vi "WS2812 Ring LED.vi"() -> ()   [LabVIEW 2017]
uses:
  IMAQCV/PIIO/Core/PIIO DIO.ctl
  IMAQCV/PIIO.lvlib
panel:
  in  "PIN":T1 items=["L1", "L2"]
  in  "Start Pixel Index":u16
  out "LED Color":u32(colorbox)
  in  "Blue":u8(slide) scale=0.0..255.0
  in  "Green":u8(slide) scale=0.0..255.0
  in  "Red":u8(slide) scale=0.0..255.0
  in  "stop":bool
  in  "Number of LEDs":u16=40
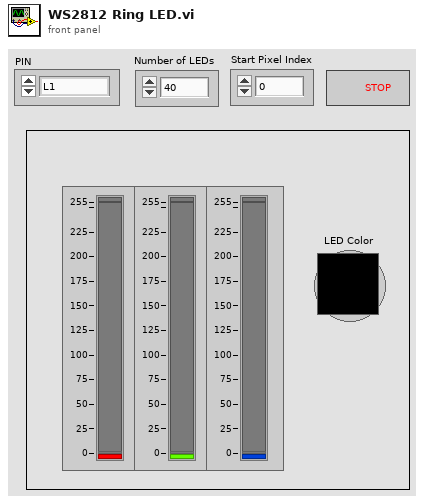
[diagram p1: front panel]
types:
  T1 = typedef "PIIO.lvlib/PIIO DIO.ctl" = u8
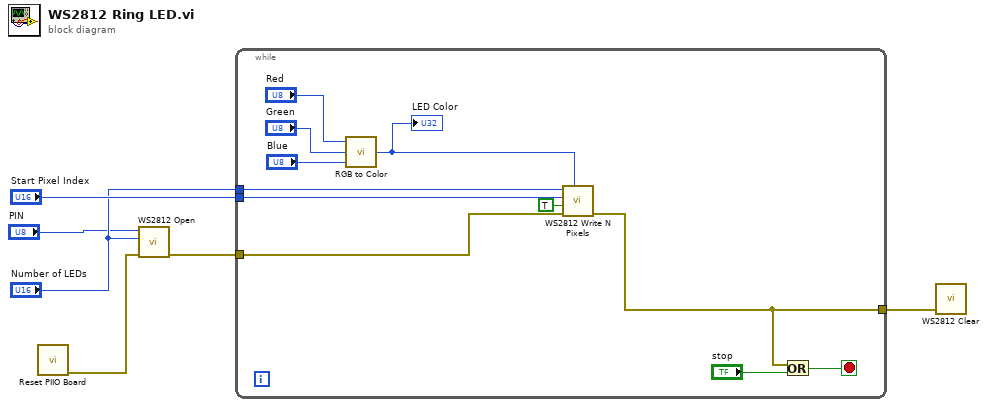
[diagram p0: block diagram]
diagram:
  n1 = call "Reset PIIO Board.vi"() -> ("error out"=w2:errorcluster)  [unwired: 11 in]
  n2 = call "WS2812 Open.vi"("Error In"=w2, "Number of LEDs"="Number of LEDs", "PIN"="PIN") -> ("Error Out"=w3:errorcluster)  [unwired: 8 in]
  n3 = while {
    tunnel: w3 -> [w9]
    tunnel: [w8] -> w4
    tunnel: "Start Pixel Index" -> [w12]
    tunnel: "Number of LEDs" -> [w11]
    stop <- w17 stop-if-true
    n4 = call <vilib>:"RGB to Color.vi"("B"="Blue", "G"="Green", "R"="Red") -> ("Color"=w10:u32)
    "LED Color" <- w10
    n5 = call "WS2812 Write N Pixels.vi"("LED Color"=w10, "Error In"=w9, "Refresh? (True)"=TRUE, "Start Pixel Index"=w12, "Number of LEDs"=w11) -> ("Error Out"=w8:errorcluster)  [unwired: 6 in]
    n6 = Or(x=w8, y="stop") -> (x .or. y?=w17:bool)
  }
  n7 = call "WS2812 Clear.vi"("Error In"=w4) -> ()  [unwired: 10 in, 1 out]
